vi "Select Pins by Device Type_wo publish id.vi"(8 "error in (no error)":errorcluster, 10 "SP4T_Pins":string[](array[string])=["RF1", "RF2", "RF3", "RF4"], 11 "USID":T1 max=15) -> (0 "error out":errorcluster, 3 "Pins_To_Test":string[](array[string]))   [LabVIEW 2013]
uses:
  Controls/USID.ctl
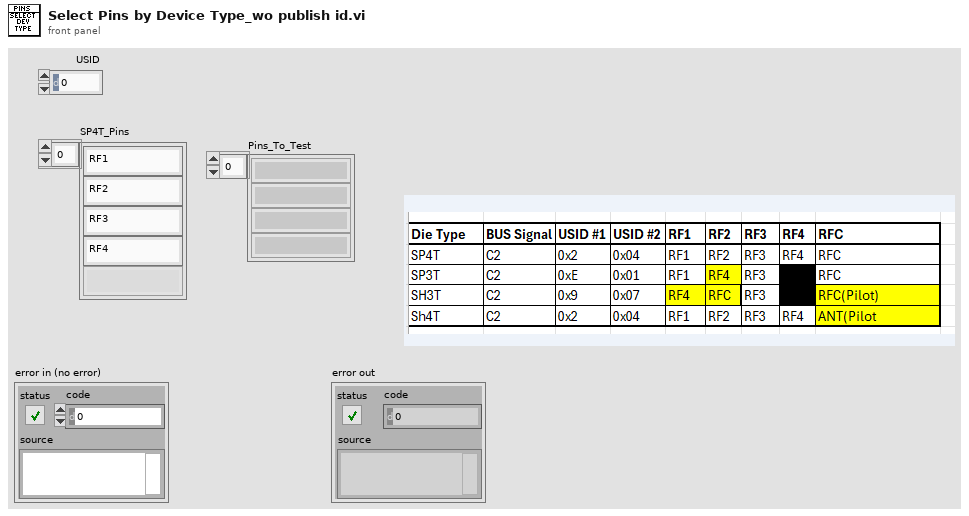
[diagram p1: front panel]
types:
  T1 = typedef "USID.ctl" = u8
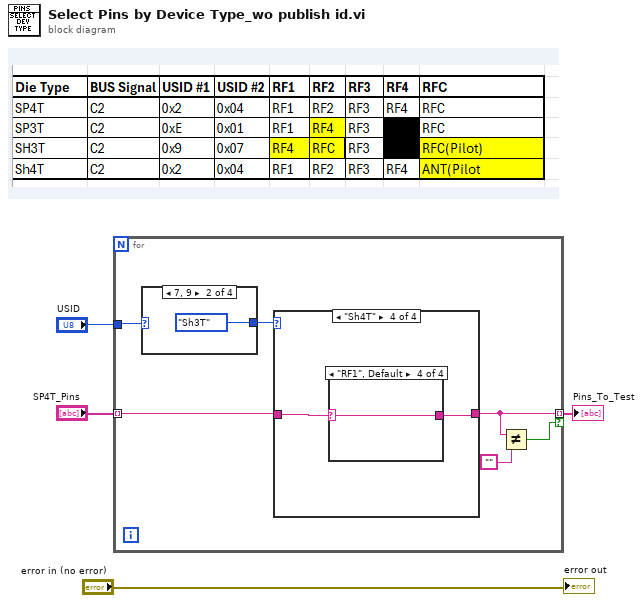
[diagram p0: block diagram]
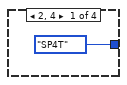
[diagram p2: hidden frame]
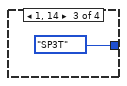
[diagram p3: hidden frame]
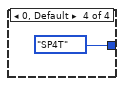
[diagram p4: hidden frame]
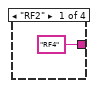
[diagram p10: hidden frame]
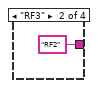
[diagram p11: hidden frame]
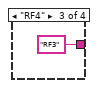
[diagram p12: hidden frame]
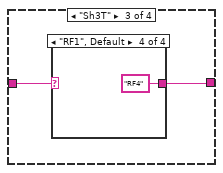
[diagram p13: hidden frame]
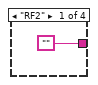
[diagram p14: hidden frame]
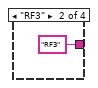
[diagram p15: hidden frame]
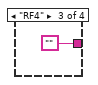
[diagram p16: hidden frame]
diagram:
  n1 = for {
    tunnel: "USID" -> [w9]
    tunnel: "SP4T_Pins" -> [w8] mode=indexing
    tunnel: [w7] -> w1 mode=indexing if=w5
    n2 = case shown="7, 9" w9 {
      tunnel: [enum16{"SP4T", "SP3T", "Sh3T", "Sh4T"}."SP4T" ("Die Type 2") enum16{"SP4T", "SP3T", "Sh3T", "Sh4T"}."Sh3T" ("Die Type 2") enum16{"SP4T", "SP3T", "Sh3T", "Sh4T"}."SP3T" ("Die Type 2") enum16{"SP4T", "SP3T", "Sh3T", "Sh4T"}."SP4T" ("Die Type 2")] -> w10
      frame 2, 4 {
      }
      frame 7, 9 {
      }
      frame 1, 14 {
      }
      frame 0, Default {
      }
    }
    n3 = case shown="\"Sh4T\"" w10 {
      tunnel: w8 -> [w16 w22 w28 w34]
      tunnel: [w15 w21 w27 w33] -> w7
      frame "SP4T", Default {
        n4 = case shown="\"RF4\"" w16 {
          selector: w16 -> [w17 w18 w19 w20]
          tunnel: [w17 w18 w19 w20] -> w15
          frame "RF2" {
          }
          frame "RF3" {
          }
          frame "RF4" {
          }
          frame "RF1", Default {
          }
        }
      }
      frame "SP3T" {
        n5 = case shown="\"RF1\", Default" w22 {
          selector: w22 -> [_ _ _ w26]
          tunnel: ["RF4" "RF2" "RF3" w26] -> w21
          frame "RF2" {
          }
          frame "RF3" {
          }
          frame "RF4" {
          }
          frame "RF1", Default {
          }
        }
      }
      frame "Sh3T" {
        n6 = case shown="\"RF1\", Default" w28 {
          tunnel: ["" "RF3" "" "RF4"] -> w27
          frame "RF2" {
          }
          frame "RF3" {
          }
          frame "RF4" {
          }
          frame "RF1", Default {
          }
        }
      }
      frame "Sh4T" {
        n7 = case shown="\"RF1\", Default" w34 {
          selector: w34 -> [w35 w36 w37 w38]
          tunnel: [w35 w36 w37 w38] -> w33
          frame "RF2" {
          }
          frame "RF3" {
          }
          frame "RF4" {
          }
          frame "RF1", Default {
          }
        }
      }
    }
    n8 = Not Equal?(x=w7, y="") -> (x != y?=w5:bool)
  }
  "Pins_To_Test" <- w1
  "error out" <- "error in (no error)"
